vi "PlaneCompass.vi"(8 "error in (no error)":errorcluster caption="error in", 11 "GPS_Ground Course":dbl=60.0 format="%#_13g") -> (0 "error out":errorcluster)   [LabVIEW 2020]
uses:
  Users/Kaitie/Desktop/LauraLabVIEW/rasppi/MultiWii_Sixpack/MultiWii_Sixpack/Sub_VIs/IMU_Functions/IMU_Data_Cluster.ctl
panel:
  in  "MultiWii Data Cluster":T1 {"Altitude abs [m]" format="%.2f"; "Baro T [°C]" format="%.1f"; "Baro P [mbara]" format="%.1f"; "GPS_coord[LON]" format="%#_9f"; "GPS_coord[LAT]" format="%#_9f"; "Altitude [m]" format="%.2f"}
  out "HeadingDigital":dbl format="%.1f"
  out "Compass 2":picture
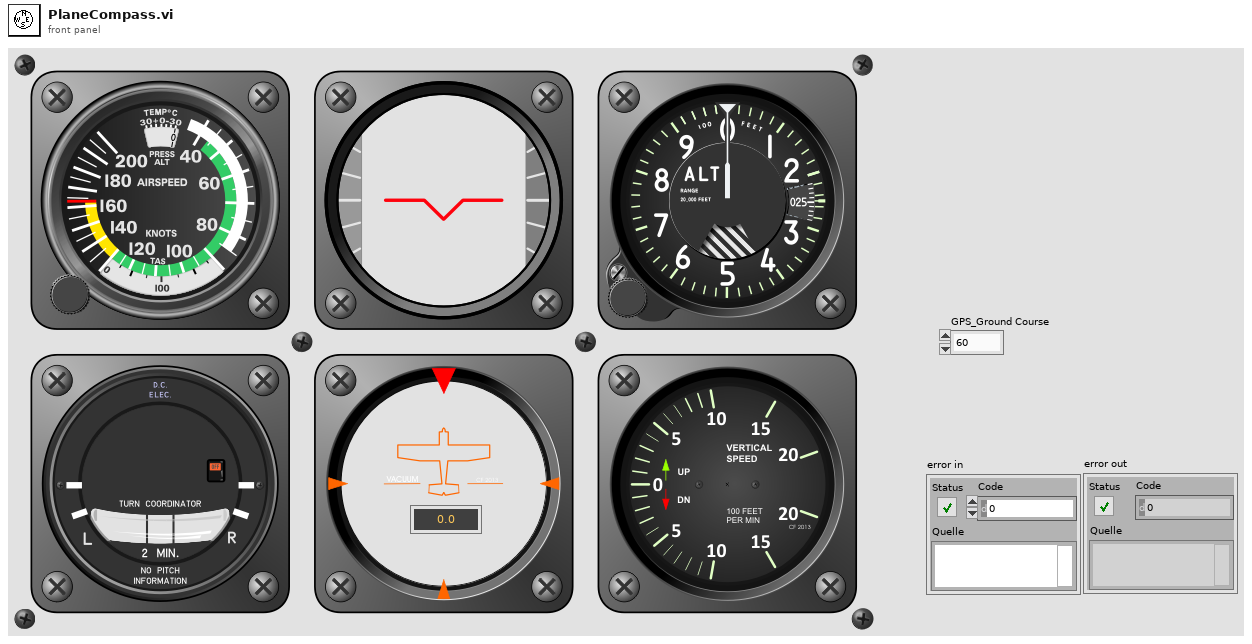
[diagram p1: front panel]
types:
  T1 = typedef "IMU_Data_Cluster.ctl" = cluster{"Firmware Revision":string, "Multitype Name":string, "Cycle Time":u16, "I²C Error Count":u16, "ACC present":bool, "Baro present":bool, "Mag Present":bool, "GPS present":bool, "Sonar present":bool, "Acc X axis (Roll)":dbl, "Acc Y axis (Pitch)":dbl, "Acc Z axis (Yaw)":dbl, "Gyro X axis (Roll)":dbl, "Gyro Y axis (Pitch)":dbl, "Gyro Z axis (Yaw)":dbl, "Mag X axis (Roll)":dbl, "Mag Y axis (Pitch)":dbl, "Mag Z axis (Yaw)":dbl, "X angle (Roll)":dbl, "Y angle (Pitch)":dbl, "Heading [°]":dbl, "Altitude [m]":dbl, "Vario":dbl, "GPS_Fix":u8, "GPS_NumSat":u8, "GPS_coord[LAT]":dbl, "GPS_coord[LON]":dbl, "GPS_Altitude":dbl, "GPS_Speed over Ground":dbl, "GPS_Ground Course":dbl, "Baro P [mbara]":dbl, "Baro T [°C]":dbl, "Altitude abs [m]":dbl}
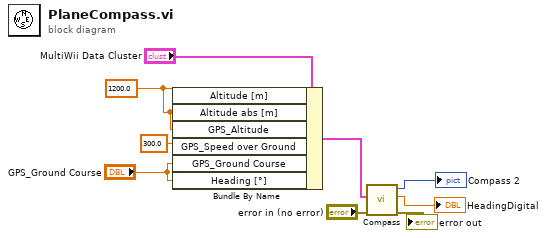
[diagram p0: block diagram]
diagram:
  w8 = 1200.0 ("Altitude [m]")
  n1 = Bundle By Name(cluster="MultiWii Data Cluster", "Altitude [m]"=w8, "Altitude abs [m]"=w8, "GPS_Altitude"=w8, "GPS_Speed over Ground"=300.0, "GPS_Ground Course"="GPS_Ground Course", "Heading [°]"="GPS_Ground Course") -> (w5:T1)
  n2 = call "Compass.vi"("error in (no error)"="error in (no error)", "MultiWii Data Cluster"=w5) -> ("error out"=→"error out":errorcluster, "Heading Digital"=→"HeadingDigital":dbl, "CompassGauge"=→"Compass 2":picture)  [unwired: 7 in]
